vi "1C SmallRCSense.vi"(10 "Wind Direction":T3=45.0 format="%05.1f", 11 "Wind Speed":dbl=1.0) -> (0 "Apparent Wind Speed":T1, 1 "Apparent Wind\nDirection":T2, 2 "Boat\nVelocity":T4, 3 "Heading":T3 format="%05.1f", 4 "Eye in the Sky":T6(plugin-control), 5 "Boat Location":T5)   [LabVIEW 2011]
doc: "TODO: finish camera interpreter\nTODO: arrange this to be easier to convert for future boats!"
uses:
  2-Think/2 Typedefs/UTM Location.ctl
  2-Think/2 Typedefs/Velocity.ctl
  2-Think/2 Typedefs/heading.ctl
  2-Think/2 Typedefs/apparent wind direction.ctl
  2-Think/2 Typedefs/apparent wind speed.ctl
  2-Think/2 Typedefs/pitch and roll.ctl
  2-Think/2 Typedefs/apparent wind.ctl
  2-Think/2 Globals/2 Global.vi
panel:
  out "Frame Rate (Hz)":dbl
  out "Apparent Wind\nin global ref frame":T4
  out "Absolute Wind":T4
  in  "Add Randomness\nTo Wind Measurement":bool
  # "TODO: upgrade speed + reliability of pattern matching"
  # "(in boat ref frame)"
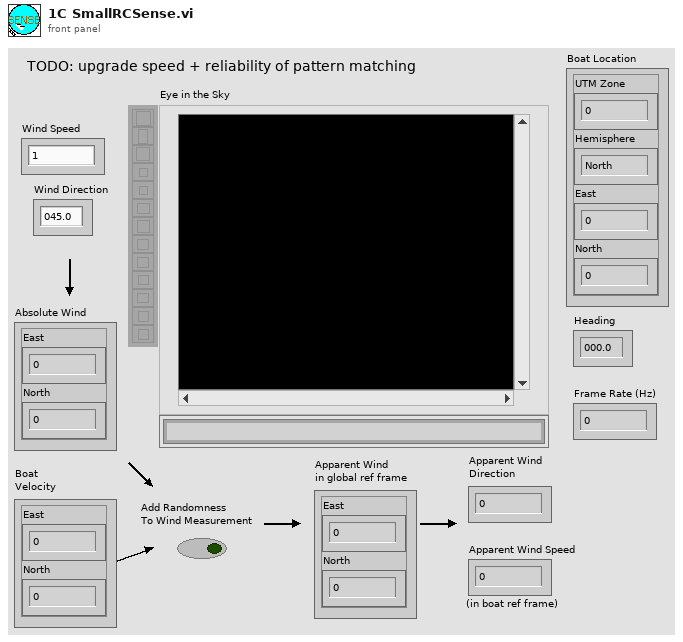
[diagram p1: front panel]
types:
  T1 = typedef "apparent wind speed.ctl" = dbl
  T2 = typedef "apparent wind direction.ctl" = dbl
  T3 = typedef "heading.ctl" = dbl
  T4 = typedef "Velocity.ctl" = cluster{"East":dbl, "North":dbl}
  T5 = typedef "UTM Location.ctl" = cluster{"UTM Zone":dbl, "Hemisphere":enum16{"North", "South"}, "East":dbl, "North":dbl}
  T6 = typedef "IMAQ Image.ctl" = refnum<image>
  T7 = typedef "pitch and roll.ctl" = cluster{"Pitch":dbl, "Roll":dbl}
  T8 = typedef "rate of turn.ctl" = dbl
  T9 = typedef "apparent wind.ctl" = cluster{"Toward Fore":dbl, "Toward Starboard":dbl}
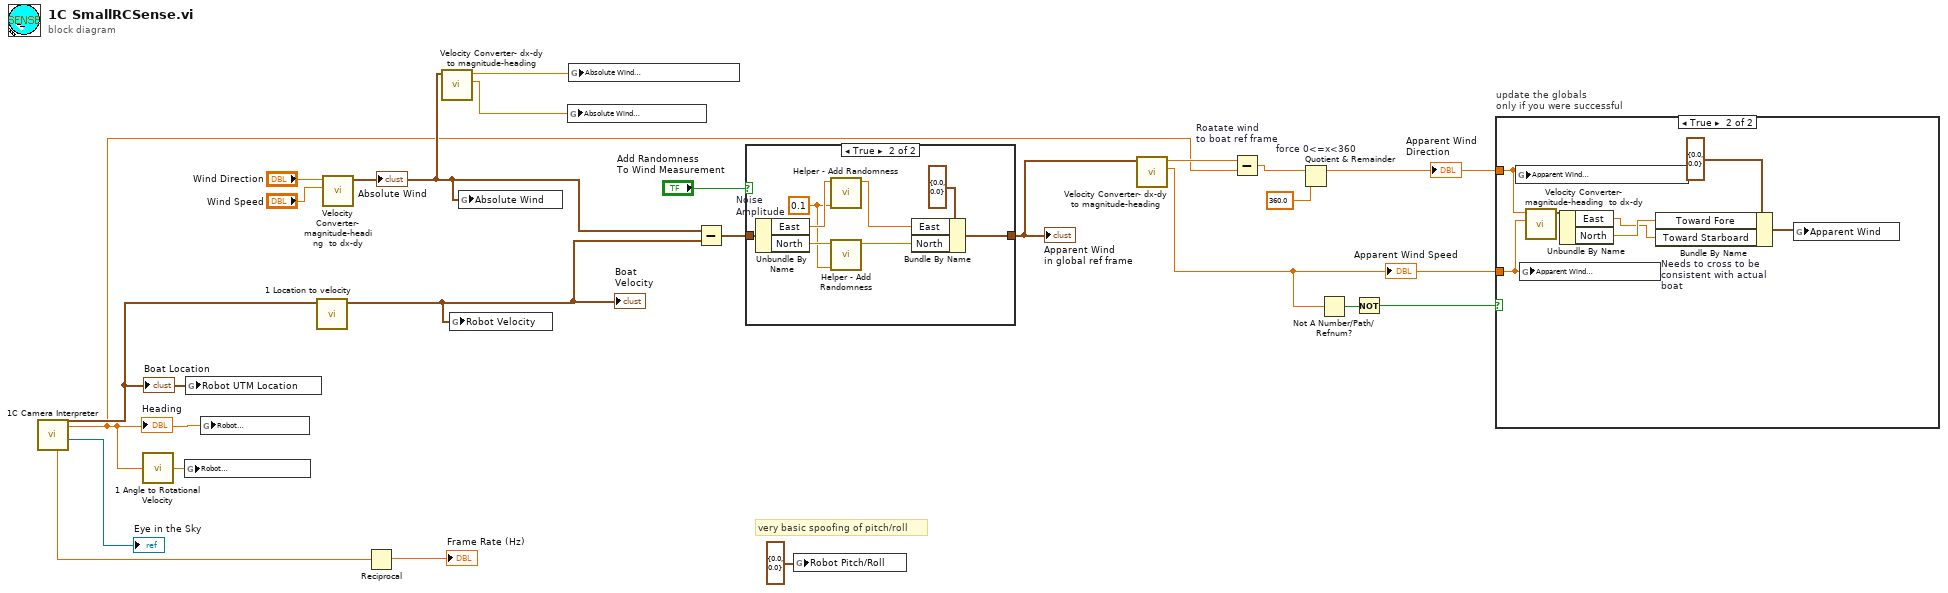
[diagram p0: block diagram]
diagram:
  # "very basic spoofing of pitch/roll"
  n1 = call "1C Camera Interpreter.vi"() -> ("Overhead Image"=→"Eye in the Sky":T6, "Heading"=w1:T3, "Boat Location"=w9:T5, "Time Elapsed (s)\nSince Last Image"=w18:dbl)  [unwired: 7 in, 1 out]
  "Boat Location" <- w9
  "Heading" <- w1
  n2 = call "1 Angle to Rotational Velocity.vi"("Robot\nHeading"=w1) -> ("Robot\nRate of Turn"=w7:T8)
  n3 = global write "2 Global.vi" "Robot\nRate of Turn"(w7) -> ()
  n4 = global write "2 Global.vi" "Robot UTM Location"(w9) -> ()
  n5 = global write "2 Global.vi" "Robot\nHeading"(w1) -> ()
  n6 = call "1 Location to velocity.vi"("Robot UTM Location"=w9) -> ("Velocity"=w8:T4)  [unwired: 10 in]
  "Boat\nVelocity" <- w8
  n7 = call "Velocity Converter- magnitude-heading  to dx-dy.vi"("Magnitude"="Wind Speed", "Heading"="Wind Direction") -> ("Vector Out"=w5:T4)  [unwired: 9 in]
  "Absolute Wind" <- w5
  n8 = Reciprocal(x=w18) -> (1/x=→"Frame Rate (Hz)":dbl)
  n9 = call "Velocity Converter- dx-dy to magnitude-heading.vi"("Vector In"=w5) -> ("Magnitude Out"=w4:dbl, "Heading Out"=w3:T3)  [unwired: 9 in]
  n10 = global write "2 Global.vi" "Robot Velocity"(w8) -> ()
  n11 = global write "2 Global.vi" "Absolute Wind"(w5) -> ()
  n12 = global write "2 Global.vi" "Absolute Wind\nSpeed"(w4) -> ()
  n13 = global write "2 Global.vi" "Absolute Wind\nDirection (º)"(w3) -> ()
  n14 = Subtract(x=w5, y=w8) -> (x-y=w12:T4)
  n15 = case shown="True" "Add Randomness\nTo Wind Measurement" {
    tunnel: [w24 w32] -> w16
    tunnel: w12 -> [w24 w31]
    frame False {
    }
    frame True {
      w26 = 0.1  # Noise Amplitude
      n16 = Unbundle By Name(w31) -> ("East"=w30:dbl, "North"=w29:dbl)
      n17 = call "Helper - Add Randomness.vi"("Amplitude\n(default 1)"=w26, "Numeric in"=w30) -> ("Numeric out"=w27:dbl)  [unwired: 9 in]
      n18 = call "Helper - Add Randomness.vi"("Amplitude\n(default 1)"=w26, "Numeric in"=w29) -> ("Numeric out"=w28:dbl)  [unwired: 9 in]
      n19 = Bundle By Name(cluster=T4 {"East"=0.0, "North"=0.0} ("Apparent Wind 2"), "East"=w27, "North"=w28) -> (w32:T4)
    }
  }
  "Apparent Wind\nin global ref frame" <- w16
  n20 = global write "2 Global.vi" "Robot Pitch/Roll"(T7 {"Pitch"=0.0, "Roll"=0.0} ("Robot Pitch/Roll")) -> ()
  n21 = call "Velocity Converter- dx-dy to magnitude-heading.vi"("Vector In"=w16) -> ("Magnitude Out"=w10:dbl, "Heading Out"=w6:T3)  [unwired: 9 in]
  "Apparent Wind Speed" <- w10
  n22 = Subtract "Roatate wind\nto boat ref frame"(x=w6, y=w1) -> (x-y=w13:T3)
  n23 = Quotient & Remainder "force 0<=x<360"(x=w13, y=T3 360.0) -> (x-y*floor(x/y)=w11:T3)  [unwired: 1 out]
  "Apparent Wind\nDirection" <- w11
  n24 = Not A Number/Path/Refnum?(number/path/refnum=w10) -> (NaN/Path/Refnum?=w15:bool)
  n25 = Not(x=w15) -> (.not. x?=w14:bool)
  n26 = case "update the globals\nonly if you were successful" shown="True" w14 {
    tunnel: w11 -> [_ w39]
    tunnel: w10 -> [_ w38]
    frame False {
    }
    frame True {
      n27 = global write "2 Global.vi" "Apparent Wind\nDirection (º)"(w39) -> ()
      n28 = global write "2 Global.vi" "Apparent Wind\nSpeed"(w38) -> ()
      n29 = call "Velocity Converter- magnitude-heading  to dx-dy.vi"("Magnitude"=w38, "Heading"=w39) -> ("Vector Out"=w37:T4)  [unwired: 9 in]
      n30 = Unbundle By Name(w37) -> ("East"=w34:dbl, "North"=w35:dbl)
      n31 = Bundle By Name "Needs to cross to be consistent with actual boat"(cluster=T9 {"Toward Fore"=0.0, "Toward Starboard"=0.0} ("Apparent Wind"), "Toward Fore"=w35, "Toward Starboard"=w34) -> (w33:T9)
      n32 = global write "2 Global.vi" "Apparent Wind"(w33) -> ()
    }
  }
